vi "Update Plot Config.vi"(8 "error in (no error)":errorcluster, 11 "HistorianCharting in":refnum<class "HistorianCharting.lvclass">) -> (0 "error out":errorcluster, 3 "HistorianCharting out":refnum<class "HistorianCharting.lvclass">)   [LabVIEW 2020, in "VolatusGUIElements.lvlib" / "HistorianCharting.lvclass"]
uses:
  HistorianCharting.lvclass
  HistorianCharting.lvclass/HistorianCharting.ctl
  Volatus/MessageQ/MessageQ.lvclass/MessageQ.ctl
  Volatus/VolatusAPI/VolatusAPI.lvclass
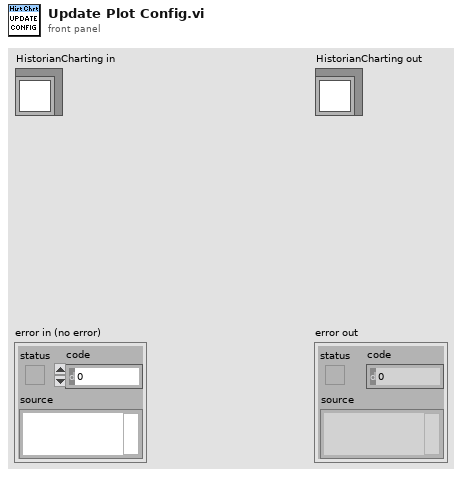
[diagram p1: front panel]
types:
  T1 = typedef "VolatusGUI.lvlib/Historian Charting Manager.lvclass/Plot Group Config.ctl" = cluster{"Name":string, "X-Axis Type":T2, "X-Axis Channel":string, "Plots":T3[], "Lock Now":bool, "Time":string, "Swap Axes":bool}
  T2 = typedef "VolatusGUI.lvlib/Historian Charting Manager.lvclass/X-Axis Type.ctl" = enum16{"Time", "Channel"}
  T3 = typedef "VolatusGUI.lvlib/Historian Charting Manager.lvclass/Plot Config.ctl" = cluster{"Channel":string, "Visible":bool, "Color":u32, "Scale":T4}
  T4 = typedef "VolatusGUI.lvlib/Historian Charting Manager.lvclass/Scale.ctl" = enum16{"Left", "Right"}
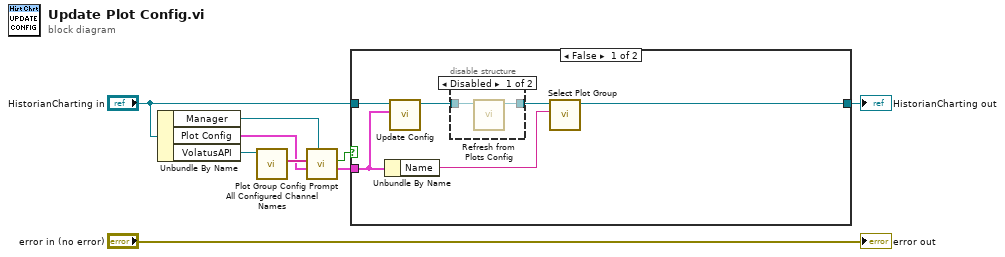
[diagram p0: block diagram]
diagram:
  n1 = Unbundle By Name("HistorianCharting in") -> ("Manager"=w1:refnum<class "MessageQ.lvclass">, "Plot Config"=w2:T1, "VolatusAPI"=w8:refnum<class "VolatusAPI.lvclass">)
  n2 = call "All Configured Channel Names.vi"("VolatusAPI in"=w8) -> ("Channel Names"=w7:string[])  [unwired: 8 in, 2 out]
  n3 = call "Plot Group Config Prompt.vi"("Manager"=w1, "Config in"=w2, "Init Available Channels"=w7) -> ("Config"=w3:T1, "Cancelled"=w6:bool)  [unwired: 7 in]
  n4 = case shown="False" w6 {
    tunnel: [w14 w19] -> w5
    tunnel: "HistorianCharting in" -> [w12 w19]
    tunnel: w3 -> [w10 _]
    frame False {
      n5 = Unbundle By Name(w10) -> ("Name"=w13:string)
      n6 = call "Update Config.vi"("Config"=w10, "HistorianCharting in"=w12) -> ("HistorianCharting out"=w11:refnum<class "HistorianCharting.lvclass">)  [unwired: 8 in, 1 out]
      n7 = disable-structure shown="Disabled" {
        disable-tunnel: w11 -> [w17 w18]
        disable-tunnel: [w16 w18] -> w15
        frame Disabled {
          n8 = call "Refresh from Plots Config.vi"("HistorianCharting in"=w17) -> ("HistorianCharting out"=w16:refnum<class "HistorianCharting.lvclass">)  [unwired: 9 in, 1 out]
        }
        frame Enabled {
        }
      }
      n9 = call "Select Plot Group.vi"("Plot Group"=w13, "HistorianCharting in"=w15) -> ("HistorianCharting out"=w14:refnum<class "HistorianCharting.lvclass">)  [unwired: 8 in, 1 out]
    }
    frame True {
    }
  }
  "HistorianCharting out" <- w5
  "error out" <- "error in (no error)"
